vi "Turn 20 Degrees Right (SubVI).vi"(8 "error in (no error)":errorcluster, 11 "Turn? Right Positive.":dbl) -> (0 "error out":errorcluster)   [LabVIEW 2017]
uses:
  <vilib>/Rock Robotics/WPI/ThirdParty/Sensors/navX/_TypeDefs/FRIC_navX_DeviceNumbersTypeDef.ctl
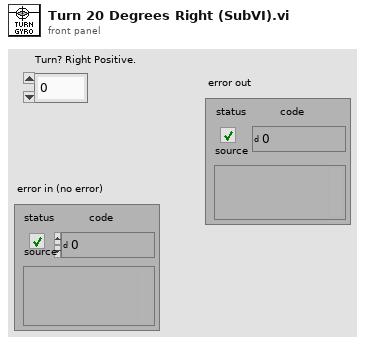
[diagram p1: front panel]
types:
  T1 = typedef "FRIC_navX_DeviceNumbersTypeDef.ctl" = enum16{"Dev0", "Dev1", "Dev2", "Dev3"}
  T2 = cluster{"Yaw":dbl, "Roll":dbl, "Pitch":dbl, "Heading":dbl, "Fused Heading":dbl}
  T3 = typedef "DriveMotors.ctl" = cluster{"MotorControlDevRef":T4, "MotorControlDevRef":T4, "MotorControlDevRef":T4, "MotorControlDevRef":T4, "MotorControlDevRef":T4, "MotorControlDevRef":T4}
  T4 = typedef "WPI_MotorControlDeviceRef.ctl" = cluster{"DeviceStatus":errorcluster, "Type":T5, "PWM":cluster{"PWM Channel":T6, "DeadBand":T7}, "CAN":cluster{"Device Number":u8, "SetOutput VI Ref":variant, "GetOutput VI Ref":variant, "Enable VI Ref":variant, "Disable VI Ref":variant, "Data":variant}, "Invert":bool, "DIO PWM":cluster{"PWM \"Enable\" Channel":T6, "DIOChannel":T8, "PWM Rate":dbl}}
  T5 = typedef "WPI_MotorControlType.ctl" = enum16{"PWM", "CAN", "DIO PWM"}
  T6 = typedef "FPGA_DIOPWMChannel.ctl" = enum8{"PWM 0", "PWM 1", "PWM 2", "PWM 3", "PWM 4", "PWM 5", "PWM 6", "PWM 7", "PWM 8", "PWM 9", "PWM MXP 0", "PWM MXP 1", "PWM MXP 2", "PWM MXP 3", "PWM MXP 4", "PWM MXP 5", "PWM MXP 6", "PWM MXP 7", "PWM MXP 8", "PWM MXP 9", "Invalid"}
  T7 = typedef "WPI_PWMDeadband.ctl" = cluster{"Name":string, "maxPositivePwm":i32, "minPositivePwm":i32, "centerPwm":i32, "maxNegativePwm":i32, "minNegativePwm":i32, "angularRange":u16}
  T8 = typedef "FPGA_DIOChannel.ctl" = enum8{"DIO 0", "DIO 1", "DIO 2", "DIO 3", "DIO 4", "DIO 5", "DIO 6", "DIO 7", "DIO 8", "DIO 9", "DIO MXP 0", "DIO MXP 1", "DIO MXP 2", "DIO MXP 3", "DIO MXP 4", "DIO MXP 5", "DIO MXP 6", "DIO MXP 7", "DIO MXP 8", "DIO MXP 9", "DIO MXP 10", "DIO MXP 11", "DIO MXP 12", "DIO MXP 13", "DIO MXP 14", "DIO MXP 15", "SPI Port CS1", "SPI Port CS2", "SPI Port CS3", "SPI Port MISO", "SPI Port MOSI", "Invalid"}
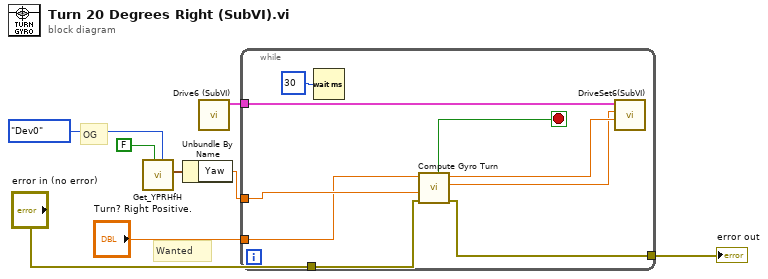
[diagram p0: block diagram]
diagram:
  # "Wanted"
  # "OG"
  n1 = call <vilib>:"Get_YPRHfH.vi"("Device Number"=FRIC_navX_DeviceNumbersTypeDef."Dev0", "Update"=FALSE) -> ("YRPHfH"=w8:T2)  [unwired: 9 in]
  n2 = Unbundle By Name(w8) -> ("Yaw"=w4:dbl)
  n3 = call "Drive6 (SubVI).vi"() -> ("DriveControlDevRef"=w5:T3)  [unwired: 11 in]
  n4 = while {
    tunnel: w5 -> [w16]
    tunnel: [w11] -> w3
    tunnel: "error in (no error)" -> [w10]
    tunnel: w4 -> [w12]
    tunnel: "Turn? Right Positive." -> [w9]
    stop <- w15 stop-if-true
    n5 = Wait (ms)(milliseconds to wait=u32 30) -> ()  [unwired: 1 out]
    n6 = call "Compute Gyro Turn.vi"("error in (no error)"=w10, "Starting Degree"=w12, "Turn? Right Positive."=w9) -> ("error out"=w11:errorcluster, "Right Drive"=w13:dbl, "Left drive"=w14:dbl, "done"=w15:bool)  [unwired: 5 in]
    n7 = call "DriveSet6(SubVI).vi"("Left"=w14, "Right"=w13, "output cluster"=w16) -> ()  [unwired: 9 in]
  }
  "error out" <- w3
